vi "Acquire_rand_num.vi"(0 "Upper limit":u64=1 min=10 max=100 step=1, 5 "Lower limit":u64=1 min=1 max=100 step=1, 11 "error in":errorcluster) -> (4 "Data":u64, 6 "Coerce upper":u64, 15 "error out":errorcluster)   [LabVIEW 2023, in "task-1.lvlib"]
doc: "Used to acquire number within an range. (the range should always be between 1 and 100)"
uses:
  <vilib>/Utility/error.llb/DialogType.ctl
  <vilib>/numeric/Random Number (Range) U64.vi
  <vilib>/numeric/sub_Random U32.vi
  task-1.lvlib
panel:
  # "The Number produced is always within 1 to 100.\nthe user can further narrow the range as they wish"
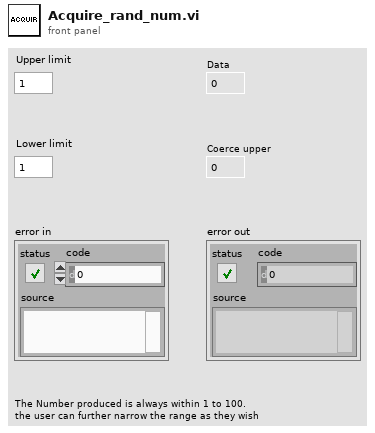
[diagram p1: front panel]
types:
  T1 = typedef "DialogType.ctl" = u16
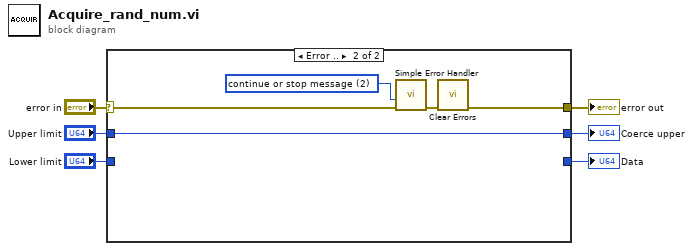
[diagram p0: block diagram]
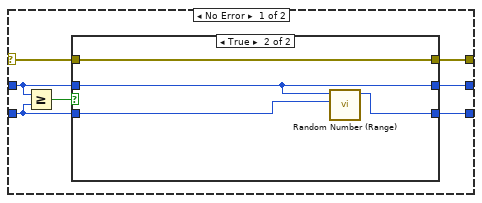
[diagram p2: hidden frame]
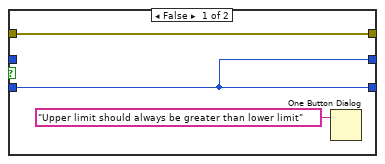
[diagram p3: hidden frame]
diagram:
  n1 = case shown="Error .." "error in" {
    selector: "error in" -> [w11 w25]
    tunnel: [w10 w22] -> w5
    tunnel: "Lower limit" -> [w12 _]
    tunnel: "Upper limit" -> [w8 w21]
    tunnel: [w7 w21] -> w2
    tunnel: [w9 _] -> w1
    frame No Error {
      n2 = Greater Or Equal?(x=w8, y=w12) -> (x >= y?=w13:bool)
      n3 = case shown="True" w13 {
        tunnel: [w15 w19] -> w9
        tunnel: w12 -> [w15 w18]
        tunnel: w8 -> [_ w17]
        tunnel: [w16 w20] -> w10
        tunnel: w11 -> [w16 w20]
        tunnel: [w15 w17] -> w7
        frame False {
          n4 = One Button Dialog(message="Upper limit should always be greater than lower limit") -> ()  [unwired: 1 in, 1 out]
        }
        frame True {
          n5 = call-poly <vilib>:"Random Number (Range).vi"("lower bound (0)"=w18, "upper bound (100)"=w17) -> ("number"=w19:u64)  [unwired: 9 in]
        }
      }
    }
    frame Error {
      w24 = T1 2 items=["no dialog", "OK message", "continue or stop message", "OK message + warnings", "continue/stop + warnings"] ("type of dialog (OK msg:1)")
      n6 = call <vilib>:"Simple Error Handler.vi"("type of dialog (OK msg:1)"=w24, "error in (no error)"=w25) -> ("error out"=w23:errorcluster)  [unwired: 3 in, 4 out]
      n7 = call <vilib>:"Clear Errors.vi"("error in (no error)"=w23) -> ("error out"=w22:errorcluster)  [unwired: 5 in, 1 out]
    }
  }
  "error out" <- w5
  "Coerce upper" <- w2
  "Data" <- w1
